vi "Start First Step.vi"(8 "error in (no error)":errorcluster, 11 "Chef Actor in":refnum<class "Chef Actor.lvclass">) -> (0 "error out":errorcluster, 3 "Chef Actor out":refnum<class "Chef Actor.lvclass">)   [LabVIEW 2024, in "Chef Actor.lvlib" / "Chef Actor.lvclass"]
uses:
  Chef Actor.lvclass
  Chef Actor.lvclass/Chef Actor.ctl
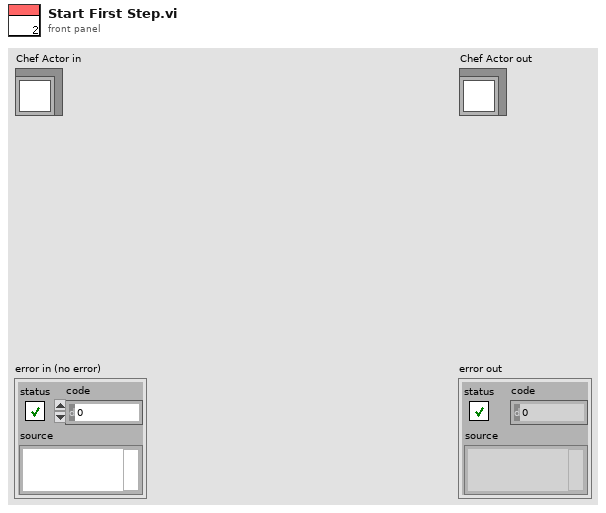
[diagram p1: front panel]
types:
  T1 = typedef "Step.ctl" = cluster{"Fire":dbl, "Duration":dbl}
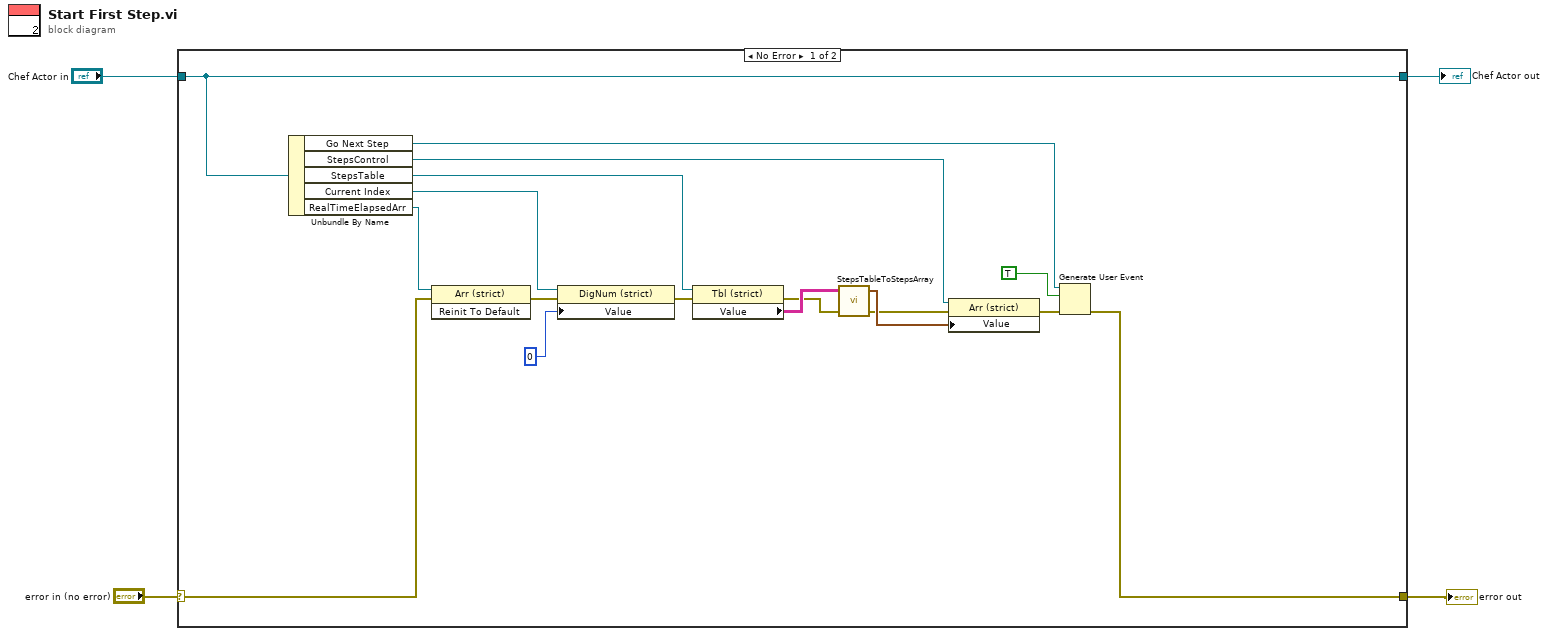
[diagram p0: block diagram]
diagram:
  n1 = case shown="No Error" "error in (no error)" {
    selector: "error in (no error)" -> [w14 w23]
    tunnel: [w10 w23] -> w3
    tunnel: [w18 w22] -> w1
    tunnel: "Chef Actor in" -> [w18 w22]
    frame No Error {
      n2 = Unbundle By Name(w18) -> ("Go Next Step"=w21:refnum<user-event>, "StepsControl"=w12:refnum<vi>, "StepsTable"=w17:refnum<vi>, "Current Index"=w8:refnum<vi>, "RealTimeElapsedArr"=w5:refnum<vi>)
      n3 = invoke class="Arr (strict)" method="Reinit To Default"(reference=w5, error in=w14) -> (error out=w6:errorcluster)  [unwired: 1 in, 2 out]
      n4 = property class="DigNum (strict)"(reference=w8, error in=w6, "Value"=0) -> (error out=w9:errorcluster)  [unwired: 1 out]
      n5 = property class="Tbl (strict)"(reference=w17, error in=w9) -> (error out=w15:errorcluster, "Value"=w16:string[][])  [unwired: 1 out]
      n6 = call "StepsTableToStepsArray.vi"("error in (no error)"=w15, "Steps Table Input"=w16) -> ("error out"=w13:errorcluster, "Steps Array Output"=w19:T1[])  [unwired: 2 in]
      n7 = property class="Arr (strict)"(reference=w12, error in=w13, "Value"=w19) -> (error out=w11:errorcluster)  [unwired: 1 out]
      n8 = Generate User Event(user event=w21, event data cluster=TRUE ("event data"), error in=w11) -> (error out=w10:errorcluster)  [unwired: 1 in, 1 out]
    }
    frame Error {
    }
  }
  "error out" <- w3
  "Chef Actor out" <- w1
